vi "practice10-21 3.vi"(8 "error in (no error)":errorcluster, 10 "baud rate":u32=1500000, 11 "VISA resource name":refnum<visa-resource-name>="COM4") -> (0 "error out":errorcluster, 3 "VISA resource name out":refnum<visa-resource-name>, 5 "F-format string":string)   [LabVIEW 2016]
uses:
  <vilib>/Instr/_visa.llb/VISA Configure Serial Port (Instr).vi
  C:/Users/TTUHEP/Documents/LabVIEW/Other Models/2010/Bin/Aerotech.A3200.dll
  Other Models/2010/Bin/Aerotech.A3200.dll
panel:
  out "x <= y?":bool
  out "Z Position":dbl
  out "controller out":refnum<k24>
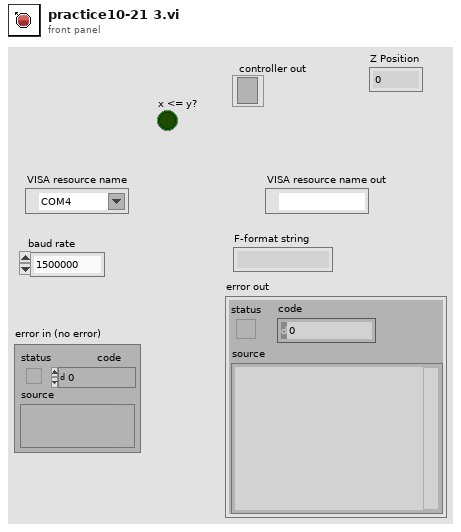
[diagram p1: front panel]
types:
  T1 = typedef "ControllerDiagPacket.ctl" = cluster{"Number of Diag Packets":i32, "Axes":T2[], "error":errorcluster}
  T2 = typedef "AxisDiagPacket.ctl" = cluster{"Axis Name":string, "Analog Input 0":dbl, "Analog Input 1":dbl, "Axis Fault (num)":i32, "Axis Fault (str)":string, "Axis Fault (bits)":cluster{"AmplifierFault":bool, "AmplifierTemperatureFault":bool, "CcwEndOfTravelLimitFault":bool, "CcwSoftwareLimitFault":bool, "CommunicationLostFault":bool, "CwEndOfTravelLimitFault":bool, "CwSoftwareLimitFault":bool, "EmergencyStopFault":bool, "EncoderFault":bool, "ExternalFault":bool, "FeedbackScalingFault":bool, "GantryMisalignFault ":bool, "HallSensorFault":bool, "InPositionTimeoutFault":bool, "InternalFault":bool, "MarkerSearchFault":bool, "MaxVelocityCommandFault":bool, "MissedInterruptFault":bool, "MotorTemperatureFault":bool, "None":bool, "OverCurrentFault":bool, "PositionErrorFault":bool, "PositionFeedbackFault":bool, "PowerSupplyFault":bool, "ProbeInputFault":bool, "SafeZoneFault":bool, "VelocityErrorFault":bool, "VelocityFeedbackFault":bool, "VoltageClampFault":bool}, "Axis Status (num)":i32, "Axis Status (str)":string, "Axis Status (bits)":cluster{"BacklashActive":bool, "CalibrationEnabled1D":bool, "CalibrationEnabled2D":bool, "CommandValid":bool, "DriveAbortPending":bool, "DrivePending":bool, "Enabling":bool, "GainMappingEnabled":bool, "GantryAligned":bool, "GantryRealigning":bool, "Homed":bool, "Homing":bool, "IFOVEnabled":bool, "JogGenerating":bool, "Jogging":bool, "JoystickControl":bool, "MasterSlaveControl":bool, "MotionBlocked":bool, "MotionClamped":bool, "MoveDone":bool, "None":bool, "NotVirtual":bool, "Profiling":bool, "Stability0":bool, "Stability1":bool, "TrajectoryFiltering":bool, "WaitDone":bool}, "Current Command":sgl, "Current Error":sgl, "Current Feedback":sgl, "Digital Inputs":i32, "Digital Outputs":i32, "Drive Status":i32, "Drive Status (str)":string, "Drive Status (bits)":cluster{"AccelerationPhase":bool, "AutofocusActive":bool, "BrakeOutput":bool, "CcwEndOfTravelLimitInput":bool, "CosineEncoderError":bool, "CurrentClamp":bool, "CwEndOfTravelLimitInput":bool, "DecelerationPhase":bool, "DualLoopActive":bool, "EmergencyStopInput":bool, "Enabled":bool, "EncoderClipping":bool, "GalvoCalibrationEnabled":bool, "GalvoPowerCorrection":bool, "HallAInput":bool, "HallBInput":bool, "HallCInput":bool, "HighResolutionMode":bool, "HomeLimitInput":bool, "InPosition":bool, "InPosition2":bool, "MarkerInput":bool, "MarkerLatch":bool, "MoveActive":bool, "NoMotorSupply":bool, "None":bool, "PowerLimiting":bool, "ProgrammingFlash":bool, "ProgrammingMXH":bool, "PSOHaltLatch":bool, "ServoControl":bool, "SineEncoderError":bool}, "Position Feedback Auxiliary":dbl, "Position Command":dbl, "Position Error":dbl, "Position Feedback":dbl, "Program Position Command":dbl, "Program Position Error":dbl, "Program Position Feedback":dbl, "Velocity Command":dbl, "Velocity Error":dbl, "Velocity Feedback":dbl}
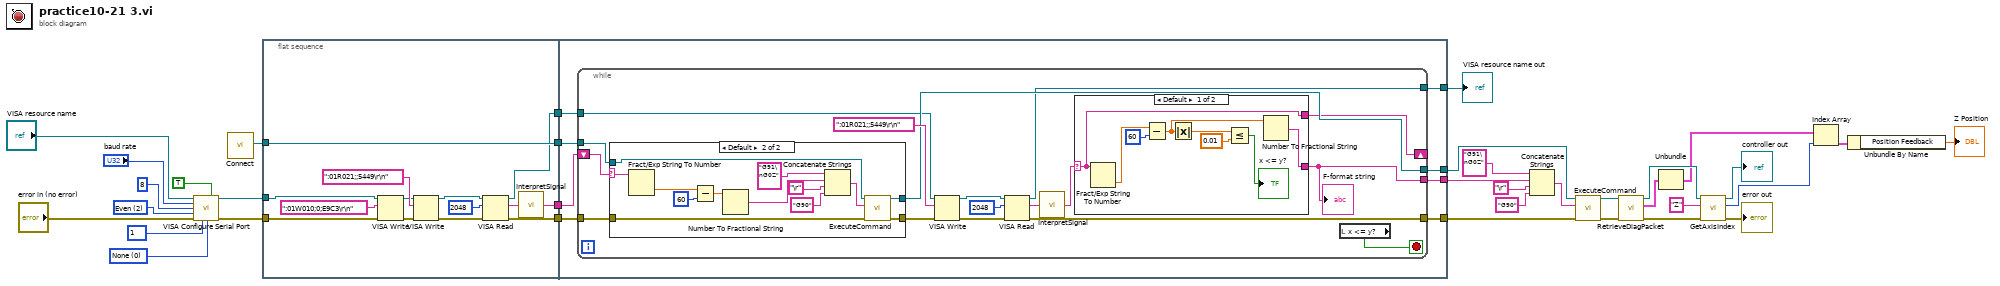
[diagram p0: block diagram]
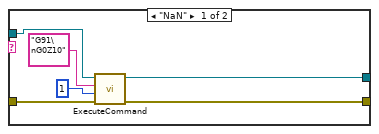
[diagram p3: hidden frame]
diagram:
  w35 = u16 0 items=["None"=0, "XON/XOFF"=1, "RTS/CTS"=2, "DTR/DSR"=4] ("flow control")
  w34 = u16 10 items=["1"=10, "1.5"=15, "2.0"=20] ("stop bits")
  w33 = u16 2 items=["None", "Odd", "Even", "Mark", "Space"] ("parity")
  n1 = call-poly "VISA Configure Serial Port"("VISA resource name"="VISA resource name", "Enable Termination\nChar (T)"=TRUE, "baud rate (9600)"="baud rate", "data bits (8)"=u16 8 ("data bits"), "parity (0:none)"=w33, "error in (no error)"="error in (no error)", "stop bits (10: 1 bit)"=w34, "flow control (0:none)"=w35) -> ("VISA resource name out"=w27:refnum<visa-resource-name>, "error out"=w26:errorcluster)  [unwired: 6 in]
  n2 = call "Connect.vi"() -> ("controller"=w24:refnum<k24>)  [unwired: 10 in, 1 out]
  n3 = flat-sequence {
    tunnel: w27 -> [w49]
    tunnel: w26 -> [w48]
    tunnel: [w46] -> w25
    tunnel: w24 -> [w46]
    tunnel: [w38] -> w3
    tunnel: [w37] -> w2
    tunnel: [w36] -> w1
    tunnel: w25 -> [w57]
    tunnel: [w56] -> w20
    tunnel: [w55] -> w6
    tunnel: [w54] -> w5
    tunnel: [w53] -> w4
    tunnel: w3 -> [w52]
    tunnel: w2 -> [w51]
    tunnel: w1 -> [w50]
    frame #0 {
      n4 = VISA Write(VISA resource name=w49, write buffer=":01W010;0;E9C3\r\n", error in (no error)=w48) -> (VISA resource name out=w40:refnum<visa-resource-name>, error out=w39:errorcluster)  [unwired: 1 out]
      n5 = VISA Write(VISA resource name=w40, write buffer=":01R021;;5449\r\n" ("Command"), error in (no error)=w39) -> (VISA resource name out=w41:refnum<visa-resource-name>, error out=w43:errorcluster)  [unwired: 1 out]
      n6 = VISA Read(VISA resource name=w41, byte count=u32 2048, error in (no error)=w43) -> (VISA resource name out=w36:refnum<visa-resource-name>, read buffer=w45:string, error out=w38:errorcluster)  [unwired: 1 out]
      n7 = call "InterpretSignal.vi"("String in"=w45) -> ("String out"=w37:string)
    }
    frame #1 {
      n8 = while {
        tunnel: w57 -> [w74]
        tunnel: [w59] -> w56
        tunnel: [w68] -> w55
        tunnel: [w67] -> w54
        tunnel: [w65] -> w53
        tunnel: w52 -> [w64]
        tunnel: w50 -> [w62]
        shift-right: [w60] -> _
        shift-left: w51 -> [w63]
        stop <- w58 stop-if-true
        n9 = case shown="Default" w63 {
          selector: w63 -> [_ w100]
          tunnel: w74 -> [w87 w92]
          tunnel: w64 -> [w86 w93]
          tunnel: [w85 w95] -> w69
          tunnel: [w84 w91] -> w68
          frame "NaN" {
            n10 = call "ExecuteCommand.vi"("error in (no error)"=w86, "taskId"=1, "Command Code"="G91\nG0Z10", "controller in"=w87) -> ("error out"=w85:errorcluster, "controller out"=w84:refnum<k24>)  [unwired: 5 in, 1 out]
          }
          frame Default {
            n11 = Fract/Exp String To Number(string=w100) -> (number=w90:dbl)  [unwired: 3 in, 1 out]
            n12 = Subtract(x=w90, y=60) -> (x-y=w101:dbl)
            n13 = Number To Fractional String(number=w101) -> (F-format string=w94:string)  [unwired: 3 in]
            n14 = Concatenate Strings("G91\nG0Z", w94, "\r", "G90") -> (w98:string)
            n15 = call "ExecuteCommand.vi"("error in (no error)"=w93, "Command Code"=w98, "controller in"=w92) -> ("error out"=w95:errorcluster, "controller out"=w91:refnum<k24>)  [unwired: 6 in, 1 out]
          }
        }
        n16 = VISA Write(VISA resource name=w62, write buffer=":01R021;;5449\r\n" ("Command"), error in (no error)=w69) -> (VISA resource name out=w73:refnum<visa-resource-name>, error out=w71:errorcluster)  [unwired: 1 out]
        n17 = VISA Read(VISA resource name=w73, byte count=u32 2048, error in (no error)=w71) -> (VISA resource name out=w65:refnum<visa-resource-name>, read buffer=w66:string, error out=w67:errorcluster)  [unwired: 1 out]
        n18 = call "InterpretSignal.vi"("String in"=w66) -> ("String out"=w61:string)
        n19 = case shown="Default" w61 {
          selector: w61 -> [w78 w83]
          tunnel: [w78 w83] -> w60
          tunnel: [w75 w83] -> w59
          frame Default {
            n20 = Fract/Exp String To Number(string=w78) -> (number=w79:dbl)  [unwired: 3 in, 1 out]
            n21 = Subtract(x=w79, y=60) -> (x-y=w77:dbl)
            n22 = Absolute Value(x=w77) -> (abs(x)=w82:dbl)
            n23 = Less Or Equal?(x=w82, y=0.01) -> (x <= y?=→"x <= y?":bool)
            n24 = Number To Fractional String(number=w77) -> (F-format string=w75:string)  [unwired: 3 in]
          }
          frame "NaN" {
          }
        }
        "F-format string" <- w59
        n25 = local read "x <= y?"() -> (w58:bool)
      }
    }
  }
  n26 = Concatenate Strings("G91\nG0Z", w20, "\r", "G90") -> (w7:string)
  n27 = call "ExecuteCommand.vi"("error in (no error)"=w5, "Command Code"=w7, "controller in"=w6) -> ("error out"=w18:errorcluster, "controller out"=w19:refnum<k24>)  [unwired: 6 in, 1 out]
  n28 = call "RetrieveDiagPacket.vi"("error in (no error)"=w18, "Controller In"=w19) -> ("error out"=w16:errorcluster, "ControllerDiagPacket"=w12:T1, "Controller Out"=w17:refnum<k24>)  [unwired: 7 in]
  n29 = Unbundle(w12) -> ("Axes"=w11:T2[])  [unwired: 2 out]
  n30 = call "GetAxisIndex.vi"("error in (no error)"=w16, "axis name"="Z", "controller in"=w17) -> ("error out"=→"error out":errorcluster, "axis index"=w10:i32, "controller out"=→"controller out":refnum<k24>)  [unwired: 6 in]
  n31 = Index Array(array=w11, index=w10) -> (element=w9:T2)
  n32 = Unbundle By Name(w9) -> ("Position Feedback"=→"Z Position":dbl)
  "VISA resource name out" <- w4
